vi "WPI_CameraSet Numeric Sensor Property.vi"(8 "error in (no error)":errorcluster, 9 "Value":i32, 10 "Property Name":string, 11 "CameraDevRef":T1) -> (0 "error out":errorcluster, 3 "CameraDevRef out":T1)   [LabVIEW 2017]
doc: "This software is licensed. Open the labview\\readme\\WPI Robotics Library Open Source License.txt file for more information."
uses:
  <vilib>/Rock Robotics/WPI/Camera/WPI_CameraDevRef.ctl
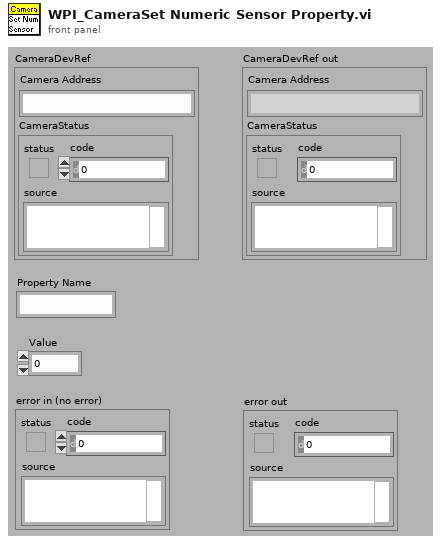
[diagram p1: front panel]
types:
  T1 = typedef "WPI_CameraDevRef.ctl" = cluster{"Camera Address":string, "CameraStatus":errorcluster}
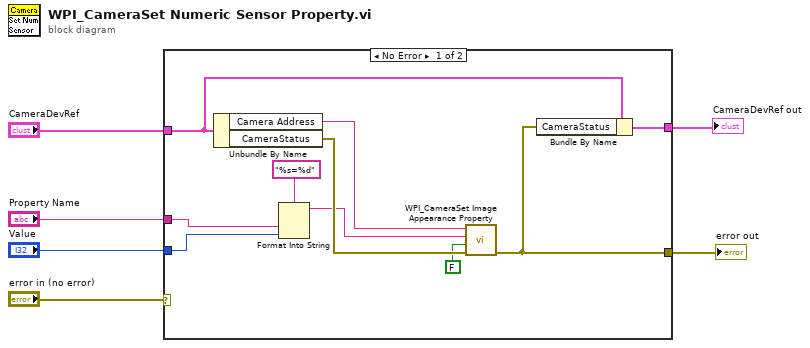
[diagram p0: block diagram]
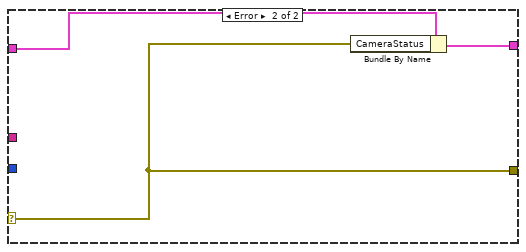
[diagram p2: hidden frame]
diagram:
  n1 = case shown="No Error" "error in (no error)" {
    selector: "error in (no error)" -> [_ w17]
    tunnel: [w11 w17] -> w6
    tunnel: "CameraDevRef" -> [w16 w18]
    tunnel: [w15 w19] -> w4
    tunnel: "Property Name" -> [w14 _]
    tunnel: "Value" -> [w13 _]
    frame No Error {
      n2 = Unbundle By Name(w16) -> ("Camera Address"=w8:string, "CameraStatus"=w10:errorcluster)
      n3 = Format Into String(format string="%s=%d", w14, w13) -> (resulting string=w9:string)  [unwired: 2 in, 1 out]
      n4 = call <vilib>:"WPI_CameraSet Image Appearance Property.vi"("error in"=w10, "Appearance"=FALSE, "Prop String"=w9, "address"=w8) -> ("error out"=w11:errorcluster)  [unwired: 7 in]
      n5 = Bundle By Name(cluster=w16, "CameraStatus"=w11) -> (w15:T1)
    }
    frame Error {
      n6 = Bundle By Name(cluster=w18, "CameraStatus"=w17) -> (w19:T1)
    }
  }
  "error out" <- w6
  "CameraDevRef out" <- w4
